vi "BuildAndLog.vi"(8 "error in (no error)":errorcluster, 10 "Command In":string, 11 "Library Builder in":refnum<class "Library Builder.lvclass">) -> (0 "error out":errorcluster, 3 "Library Builder out":refnum<class "Library Builder.lvclass">)   [LabVIEW 2020, in "Library Builder.lvclass"]
uses:
  Library Builder.lvclass
  Library Builder.lvclass/Library Builder.ctl
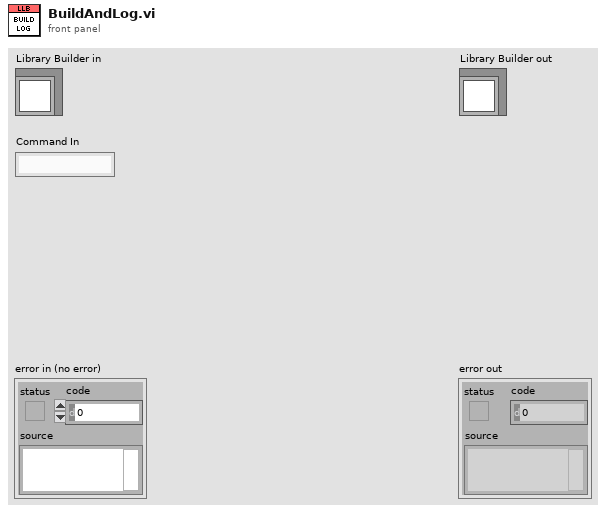
[diagram p1: front panel]
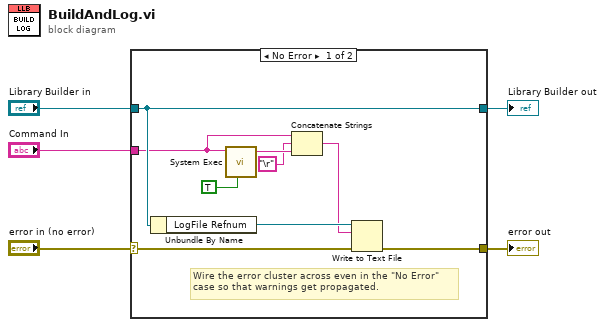
[diagram p0: block diagram]
diagram:
  n1 = case shown="No Error" "error in (no error)" {
    selector: "error in (no error)" -> [w11 w16]
    tunnel: [w10 w16] -> w4
    tunnel: [w13 w15] -> w2
    tunnel: "Library Builder in" -> [w13 w15]
    tunnel: "Command In" -> [w9 _]
    frame No Error {
      # "Wire the error cluster across even in the \"No Error\"\ncase so that warnings get propagated."
      n2 = Unbundle By Name(w13) -> ("LogFile Refnum"=w12:refnum<file>)
      n3 = call <vilib>:"System Exec.vi"("run minimized? (F)"=TRUE, "command line"=w9) -> ("standard output"=w7:string)  [unwired: 6 in, 3 out]
      n4 = Concatenate Strings(w9, "\r", w7) -> (w8:string)
      n5 = Write to Text File(file (use dialog)=w12, text=w8, error in=w11) -> (error out=w10:errorcluster)  [unwired: 1 in, 2 out]
    }
    frame Error {
    }
  }
  "error out" <- w4
  "Library Builder out" <- w2
